vi "ep_EN50160 Basic Statistical Evaluation (2D).vi"(0 "data":dbl[][](array[numeric]), 1 "evaluated data":enum16{"all data", "data without flag"}(ring), 5 "data flags":bool[][](array[boolean]), 7 "EN50160 limits":T2={"upper limit"=110.0, "lower limit"=90.0, "required percentage to be in limits"=95.0}, 11 "error in (no error)":errorcluster) -> (4 "EN50160 results":T1(array[cluster]), 10 "passed?":bool, 15 "error out":errorcluster)   [LabVIEW 2011, in "NI_EP_Power Quality.lvlib"]
uses:
  <vilib>/addons/Electrical Power/PQ/NI_EP_Power Quality.lvlib
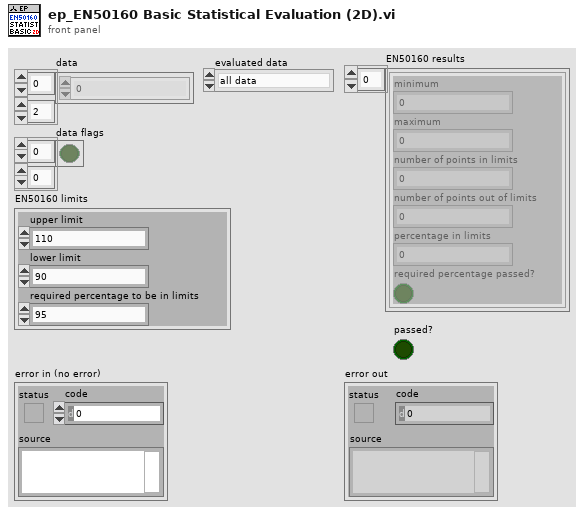
[diagram p1: front panel]
types:
  T1 = cluster{"minimum":dbl, "maximum":dbl, "number of points in limits":u32, "number of points out of limits":u32, "percentage in limits":dbl, "required percentage passed?":bool}[]
  T2 = cluster{"upper limit":dbl, "lower limit":dbl, "required percentage to be in limits":dbl}
  T3 = cluster{"minimum":dbl, "maximum":dbl, "number of points in limits":u32, "number of points out of limits":u32, "percentage in limits":dbl, "required percentage passed?":bool}
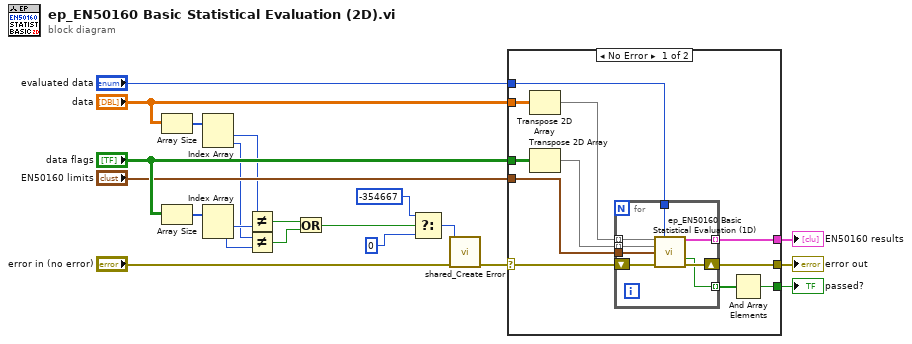
[diagram p0: block diagram]
diagram:
  n1 = Array Size(array="data") -> (size(s)=w15:i32[])
  n2 = Array Size(array="data flags") -> (size(s)=w14:i32[])
  n3 = Index Array(array=w15) -> (element #1=w12:i32, element #2=w9:i32)  [unwired: 2 in]
  n4 = Index Array(array=w14) -> (element #1=w13:i32, element #2=w10:i32)  [unwired: 2 in]
  n5 = Not Equal?(x=w12, y=w13) -> (x != y?=w7:bool)
  n6 = Not Equal?(x=w9, y=w10) -> (x != y?=w8:bool)
  n7 = Or(x=w7, y=w8) -> (x .or. y?=w6:bool)
  n8 = Select(t=-354667 ("error code (0)"), s=w6, f=0 ("error code (0)")) -> (s? t:f=w3:i32)
  n9 = call <vilib>:"shared_Create Error.vi"("error in (no error)"="error in (no error)", "error code (0)"=w3) -> ("error out"=w2:errorcluster)  [unwired: 9 in]
  n10 = case shown="No Error" w2 {
    selector: w2 -> [w27 w41]
    tunnel: "evaluated data" -> [w28 _]
    tunnel: "data" -> [w32 _]
    tunnel: "data flags" -> [w31 _]
    tunnel: [w26 w41] -> w20
    tunnel: [w29 _] -> w19
    tunnel: "EN50160 limits" -> [w30 _]
    tunnel: [w24 _] -> w11
    frame No Error {
      n11 = Transpose 2D Array(2D array=w32) -> (transposed array=w22:dbl[][])
      n12 = Transpose 2D Array(2D array=w31) -> (transposed array=w23:bool[][])
      n13 = for {
        tunnel: w22 -> [w40] mode=indexing
        tunnel: w23 -> [w39] mode=indexing
        tunnel: w30 -> [w38]
        shift-right: [w36] -> w26
        shift-left: w27 -> [w35]
        tunnel: [w37] -> w29 mode=indexing
        tunnel: w28 -> [w34]
        tunnel: [w33] -> w25 mode=indexing
        n14 = call <vilib>:"ep_EN50160 Basic Statistical Evaluation (1D).vi"("data"=w40, "evaluated data"=w34, "data flags"=w39, "EN50160 limits"=w38, "error in (no error)"=w35) -> ("EN50160 result"=w37:T3, "passed?"=w33:bool, "error out"=w36:errorcluster)  [unwired: 8 in]
      }
      n15 = And Array Elements(Boolean array=w25) -> (logical AND=w24:bool)
    }
    frame Error {
    }
  }
  "EN50160 results" <- w19
  "error out" <- w20
  "passed?" <- w11
